vi "ROI Build.vi"(8 "Angle":dbl, 9 "input cluster":T2, 10 "Centre Y":dbl, 11 "Centre X":dbl) -> (3 "ROI Descriptor":T1 {"Contours"."Type" items=["No Selection", "Point", "Line", "Rectangle", "Oval", "Polygon", "Freehand Region", "Annulus", "Unused2", "Unused3", "Broken Line", "Freehand Line", "Rotated Rectangle"]})   [LabVIEW 2019, in "Algorithm.lvclass"]
uses:
  FrameworkOverrides/Algorithm.lvclass
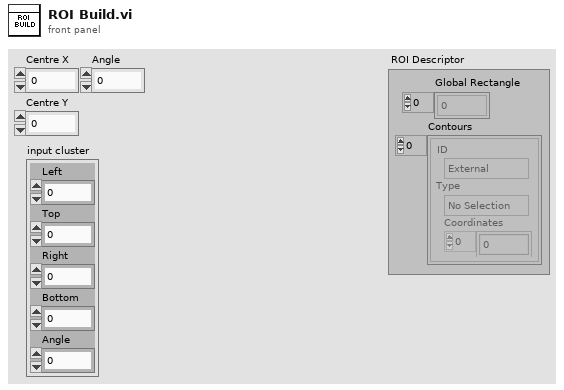
[diagram p1: front panel]
types:
  T1 = typedef "ROI Descriptor" = cluster{"Global Rectangle":i32[], "Contours":cluster{"ID":enum32{"External", "Internal"}, "Type":u32, "Coordinates":i32[]}[]}
  T2 = cluster{"Left":dbl, "Top":dbl, "Right":dbl, "Bottom":dbl, "Angle":dbl}
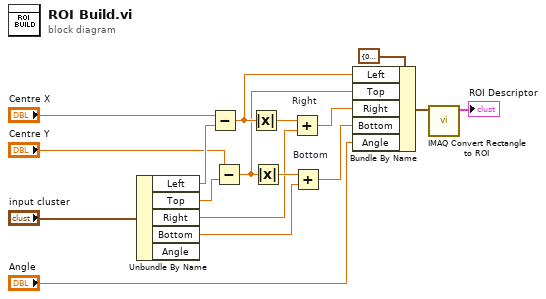
[diagram p0: block diagram]
diagram:
  n1 = Unbundle By Name("input cluster") -> ("Left"=w10:dbl, "Top"=w9:dbl, "Right"=w8:dbl, "Bottom"=w7:dbl)  [unwired: 1 out]
  n2 = Subtract(x="Centre X", y=w10) -> (x-y=w14:dbl)
  n3 = Subtract(x="Centre Y", y=w9) -> (x-y=w13:dbl)
  n4 = Absolute Value(x=w14) -> (abs(x)=w17:dbl)
  n5 = Absolute Value(x=w13) -> (abs(x)=w16:dbl)
  n6 = Add "Right"(x=w17, y=w8) -> (x+y=w12:dbl)
  n7 = Add "Bottom"(x=w16, y=w7) -> (x+y=w11:dbl)
  n8 = Bundle By Name(cluster=T2 {"Left"=0.0, "Top"=0.0, "Right"=0.0, "Bottom"=0.0, "Angle"=0.0} ("input cluster"), "Left"=w14, "Top"=w13, "Right"=w12, "Bottom"=w11, "Angle"="Angle") -> (w6:T2)
  n9 = call "IMAQ Convert Rectangle to ROI"("Rectangle"=w6) -> ("ROI Descriptor"=→"ROI Descriptor":T1)  [unwired: 8 in, 1 out]
